vi "GetWindowDC.vi"(11 "WindowHandle":u32) -> (3 "HDC":u32)   [LabVIEW 2018]
uses:
  user32.dll
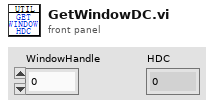
[diagram p1: front panel]
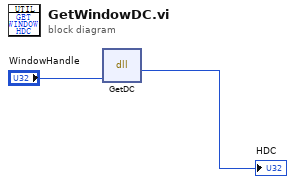
[diagram p0: block diagram]
diagram:
  n1 = dll-call lib="user32.dll" fn="GetDC"("WindowHandle"="WindowHandle") -> ("返回类型"=→"HDC":u32)  [unwired: 4 in, 2 out]
